vi "Do.vi"(8 "error in (no error)":errorcluster, 10 "Actor in":refnum<class "Actor.lvclass">, 11 "UpdateMeasurementDirectory Msg":refnum<class "UpdateMeasurementDirectory Msg.lvclass">) -> (0 "error out":errorcluster, 2 "Actor out":refnum<class "Actor.lvclass">)   [LabVIEW 2019, in "ViewerManager.lvlib" / "UpdateMeasurementDirectory Msg.lvclass"]
doc: "This VI delivers the message to the actor by calling the appropriate method(s) on the actor."
uses:
  UpdateMeasurementDirectory Msg.lvclass
  <vilib>/ActorFramework/Actor/Actor.lvclass
  UpdateMeasurementDirectory Msg.lvclass/UpdateMeasurementDirectory Msg.ctl
  ViewerManager/ViewerManager.lvclass
  C:/Program Files (x86)/National Instruments/LabVIEW 2019/vi.lib/ActorFramework/Actor/Actor.lvclass
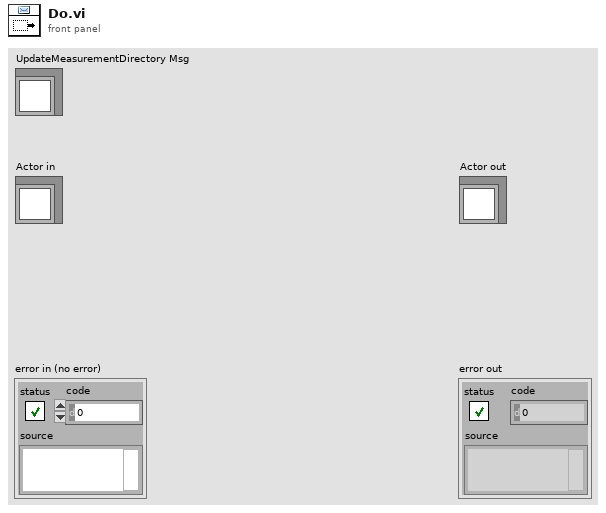
[diagram p1: front panel]
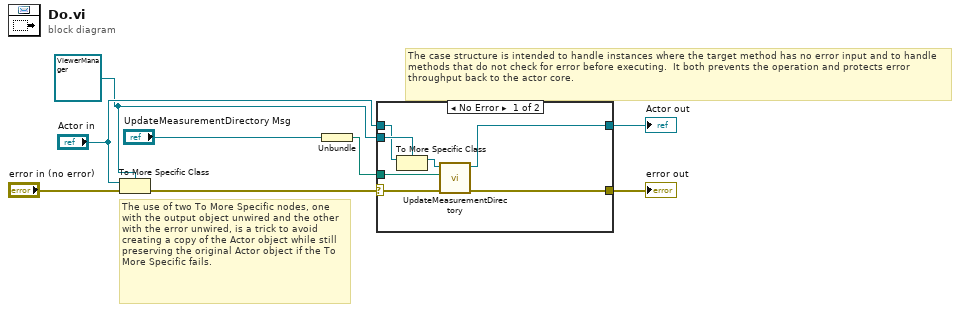
[diagram p0: block diagram]
diagram:
  w2 = refnum<class "ViewerManager.lvclass"> refnum ("Actor in")
  # "The use of two To More Specific nodes, one with the output object unwired and the other with the error unwired, is a trick to avoid creating a copy of the Actor object while still preserving the original Actor object if the To More Specific fails."
  # "The case structure is intended to handle instances where the target method has no error input and to handle methods that do not check for error before executing.  It both prevents the operation and protects error throughput back to the actor core."
  n1 = To More Specific Class(target class=w2, reference="Actor in", error in="error in (no error)") -> (error out=w6:errorcluster)  [unwired: 1 out]
  n2 = Unbundle("UpdateMeasurementDirectory Msg") -> (w1:path)
  n3 = case shown="No Error" w6 {
    selector: w6 -> [w15 w17]
    tunnel: [w11 w17] -> w5
    tunnel: [w9 w16] -> w4
    tunnel: "Actor in" -> [w12 w16]
    tunnel: w2 -> [w13 _]
    tunnel: w1 -> [w10 _]
    frame No Error {
      n4 = To More Specific Class(target class=w13, reference=w12) -> (specific class reference=w14:refnum<class "ViewerManager.lvclass">)  [unwired: 1 in, 1 out]
      n5 = call "UpdateMeasurementDirectory.vi"("error in (no error)"=w15, "Measurement Directory"=w10, "ViewerManager in"=w14) -> ("error out"=w11:errorcluster, "ViewerManager out"=w9:refnum<class "ViewerManager.lvclass">)  [unwired: 7 in]
    }
    frame Error {
      # "If type check fails, pass the original object out again."
    }
  }
  "error out" <- w5
  "Actor out" <- w4
